vi "EntradaAnalogica.vi"() -> ()   [LabVIEW 2023]
uses:
  <vilib>/Instr/_visa.llb/VISA Configure Serial Port (Instr).vi
panel:
  out "Waveform Chart":dbl(graph)
  out "Tank":dbl(slide) scale=0.0..3.3
  out "Gauge":dbl(knob) scale=0.0..10.0
  out "Valor analogico":dbl
  in  "stop":bool
  in  "VISA resource name":refnum<visa-resource-name>
  out "Meter":ext(knob) scale=0.0..3.3
  # "Medidor de voltaje"
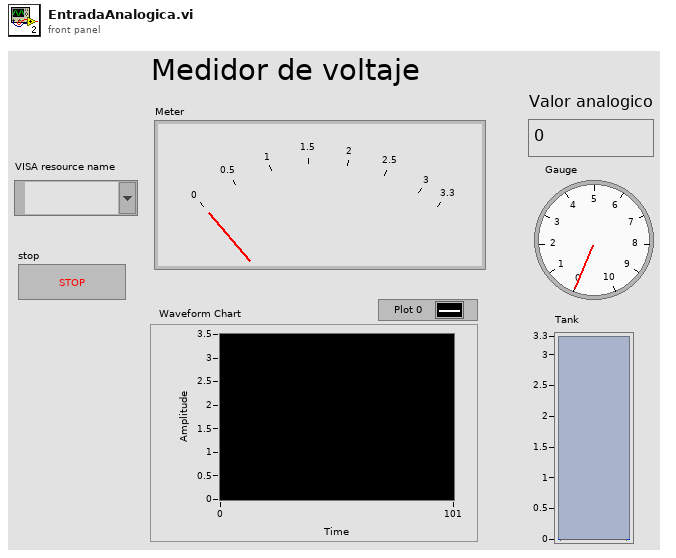
[diagram p1: front panel]
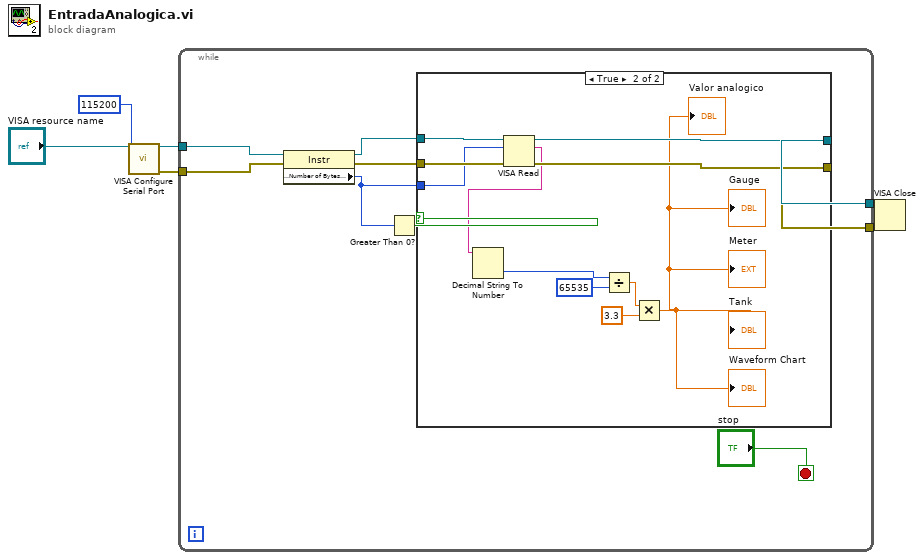
[diagram p0: block diagram]
diagram:
  n1 = call-poly "VISA Configure Serial Port"("VISA resource name"="VISA resource name", "baud rate (9600)"=u32 115200) -> ("VISA resource name out"=w4:refnum<visa-resource-name>, "error out"=w3:errorcluster)  [unwired: 12 in]
  n2 = while {
    tunnel: w4 -> [w14]
    tunnel: w3 -> [w13]
    tunnel: [w10] -> w2
    tunnel: [w9] -> w1
    stop <- "stop" stop-if-true
    n3 = property class="Instr"(reference=w14, error in=w13) -> (reference out=w12:refnum<visa-resource-name>, error out=w11:errorcluster, "Serial Settings:Number of Bytes at Serial Port"=w7:u32)
    n4 = Greater Than 0?(x=w7) -> (x > 0?=w8:bool)
    n5 = case shown="True" w8 {
      tunnel: w12 -> [w17 w28]
      tunnel: w11 -> [w16 w27]
      tunnel: [w17 w26] -> w10
      tunnel: [w16 w25] -> w9
      tunnel: w7 -> [_ w23]
      frame False {
      }
      frame True {
        n6 = VISA Read(VISA resource name=w28, byte count=w23, error in (no error)=w27) -> (VISA resource name out=w26:refnum<visa-resource-name>, read buffer=w24:string, error out=w25:errorcluster)  [unwired: 1 out]
        n7 = Decimal String To Number(string=w24) -> (number=w22:i32)  [unwired: 2 in, 1 out]
        n8 = Divide(x=w22, y=65535) -> (x/y=w20:dbl)
        n9 = Multiply(x=w20, y=3.3) -> (x*y=→"Meter" →"Valor analogico" →"Tank" →"Gauge" →"Waveform Chart":dbl)
      }
    }
  }
  n10 = VISA Close(VISA resource name=w2, error in (no error)=w1) -> ()  [unwired: 1 out]
